vi "Generate Address.vi"(8 "error in (no error)":errorcluster, 11 "10-Bit in":refnum<class "10-Bit.lvclass">) -> (0 "error out":errorcluster, 3 "10-Bit out":refnum<class "10-Bit.lvclass">)   [LabVIEW 2020, in "10-Bit.lvclass"]
uses:
  10-Bit.lvclass
  Parent/Addressing Mode.lvclass
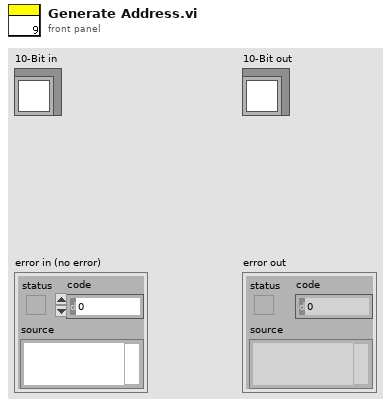
[diagram p1: front panel]
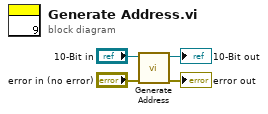
[diagram p0: block diagram]
diagram:
  n1 = call-parent "Generate Address.vi"("error in (no error)"="error in (no error)", "Addressing Mode in"="10-Bit in") -> ("error out"=→"error out":errorcluster, "Addressing Mode out"=→"10-Bit out":refnum<class "10-Bit.lvclass">)  [unwired: 8 in]
